vi "ScanPLC_Config.vi"(9 "PLC Connection Array":T2(array[cluster]) {"MemoryType" items=["CR (Control Relay)", "MR (Internal Auxiliary Relay)", "VB (Work Relay)", "LR (Latch Relay)", "B (Link Relay)", "R (Relay)", "DM (Data Memory)", "EM (Extended Data Memory)", "FM (File Register 1)", "ZF (FIle Register 2)", "W (Link Register)", "TM (Temporary Data Memory)", "Z (Index Register)", "T (Timer)", "TC (Timer (Counter Value))", "TS (Timer Set Value)", "C (Counter)", "CC (Counter (Counter Value))", "CS (Counter (Set Value))", "CTH (High Speed Counter)", "CTC (High Speed Counter Comparator (Set Value))", "AT (Digital Trimmer)", "CM (Control Memory)", "VM (Work Memory)"]; "PLC Type" items=["Keyence", "Allen Bradley", "Mitsubishi", "Panasonic", "Siemens"]}, 11 "Parameter":string) -> (1 "ConnectionInformation":T1)   [LabVIEW 2017]
panel:
  out "Index":i32
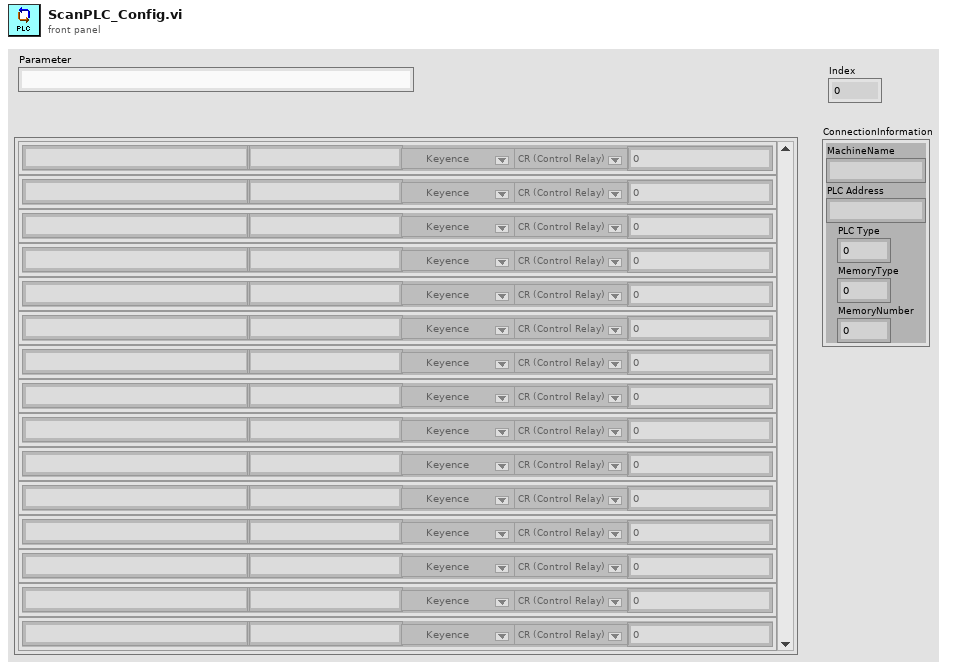
[diagram p1: front panel]
types:
  T1 = cluster{"MachineName":string, "PLC Address":string, "PLC Type":u16, "MemoryType":u16, "MemoryNumber":i32}
  T2 = cluster{"MachineName":string, "PLC Address":string, "PLC Type":u16, "MemoryType":u16, "MemoryNumber":i32}[]
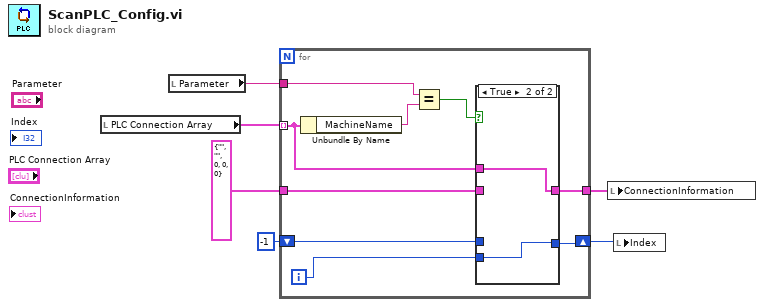
[diagram p0: block diagram]
diagram:
  n1 = local read "PLC Connection Array"() -> (w5:T2)
  n2 = local read "Parameter"() -> (w6:string)
  n3 = for {
    tunnel: w5 -> [w7] mode=indexing
    tunnel: w6 -> [w14]
    shift-right: [w10] -> w3
    shift-left: -1 -> [w12]
    tunnel: T1 {"MachineName"="", "PLC Address"="", "PLC Type"=0, "MemoryType"=0, "MemoryNumber"=0} ("ConnectionInformation") -> [w9]
    tunnel: [w8] -> w1
    i -> [w11]
    n4 = Unbundle By Name(w7) -> ("MachineName"=w15:string)
    n5 = Equal?(x=w14, y=w15) -> (x = y?=w13:bool)
    n6 = case shown="True" w13 {
      tunnel: w12 -> [w17 _]
      tunnel: [w17 w19] -> w10
      tunnel: w11 -> [_ w19]
      tunnel: w9 -> [w16 _]
      tunnel: [w16 w18] -> w8
      tunnel: w7 -> [_ w18]
      frame False {
      }
      frame True {
      }
    }
  }
  n7 = local write "ConnectionInformation"(w1) -> ()
  n8 = local write "Index"(w3) -> ()
